vi "Get New Level.vi"(8 "error in (no error)":cluster{"状态":bool, "代码":i32, "源":string} caption="错误输入（无错误）", 11 "水位控制器输入":refnum<class "Level Controller.lvclass">) -> (0 "error out":cluster{"状态":bool, "代码":i32, "源":string} caption="错误输出", 2 "水位":dbl, 3 "水位控制器输出":refnum<class "Level Controller.lvclass">)   [LabVIEW 2015, in "Level Controller.lvlib" / "Level Controller.lvclass"]
doc: "该VI设定水位控制器负责监控的变量。该VI被调用时将返回变量的当前值。子类中必须对该方法进行重写。"
uses:
  Level Controller.lvclass
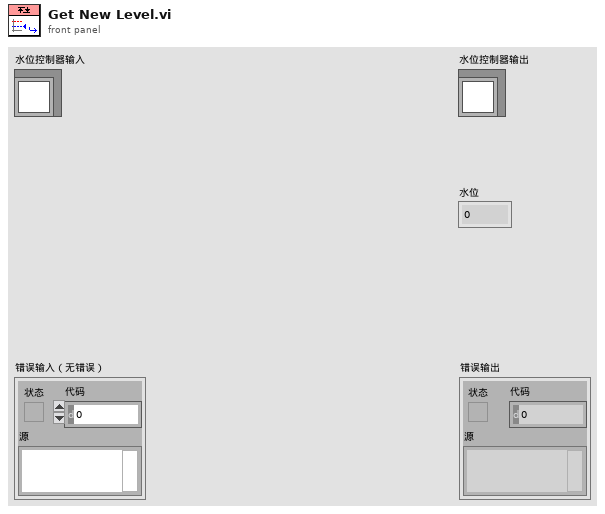
[diagram p1: front panel]
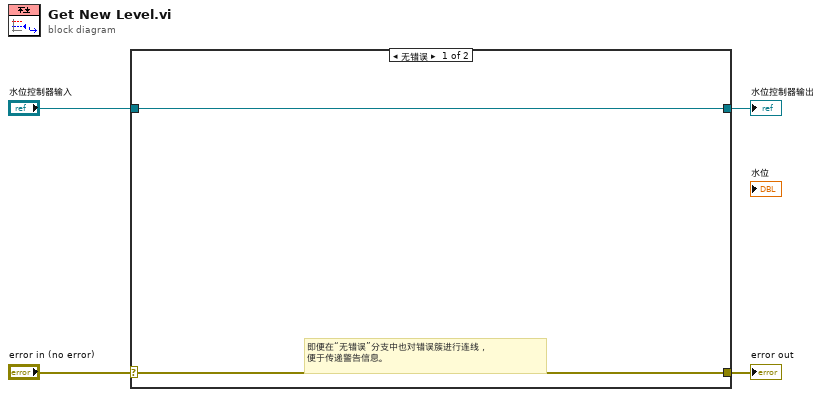
[diagram p0: block diagram]
diagram:
  n1 = case shown="无错误" "error in (no error)" {
    selector: "error in (no error)" -> [w5 w8]
    tunnel: [w5 w8] -> w3
    tunnel: [w6 w7] -> w1
    tunnel: "水位控制器输入" -> [w6 w7]
    frame No Error {
      # "即便在“无错误”分支中也对错误簇进行连线，\n便于传递警告信息。"
    }
    frame Error {
    }
  }
  "error out" <- w3
  "水位控制器输出" <- w1
